vi "LVClass_HasoData dtor.vi"(0 "HasoData in":refnum<class "HasoData.lvclass">, 11 "error in (no error)":errorcluster) -> (4 "HasoData out":refnum<class "HasoData.lvclass">, 15 "error out":errorcluster)   [LabVIEW 2020, in "HasoData.lvclass"]
doc: "HasoData destructor.\n\n--------------------------------------------------------------------------------\n\n<B>HasoDataIn </B> : Pointer to HasoData object.\n<B>HasoDataOut </B> : Pointer to HasoData object.\n<B>ErrorIn </B> : Error\n<B>ErrorOut </B> : Error\n\n--------------------------------------------------------------------------------"
uses:
  HasoData.lvclass
  HasoData.lvclass/HasoData.ctl
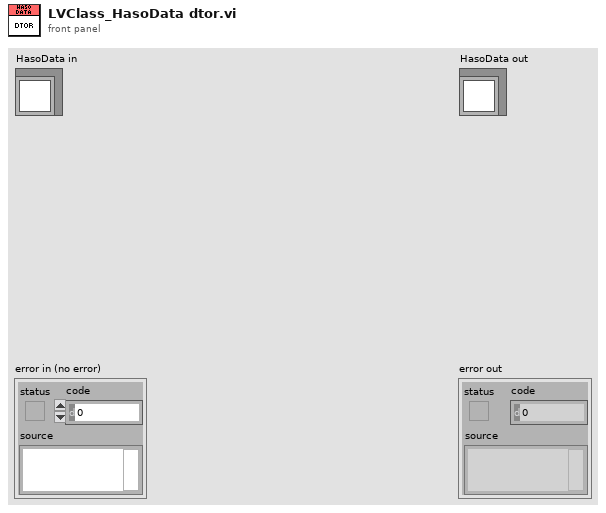
[diagram p1: front panel]
types:
  T1 = typedef "Handle creation.ctl" = enum16{"By ctor", "By write function"}
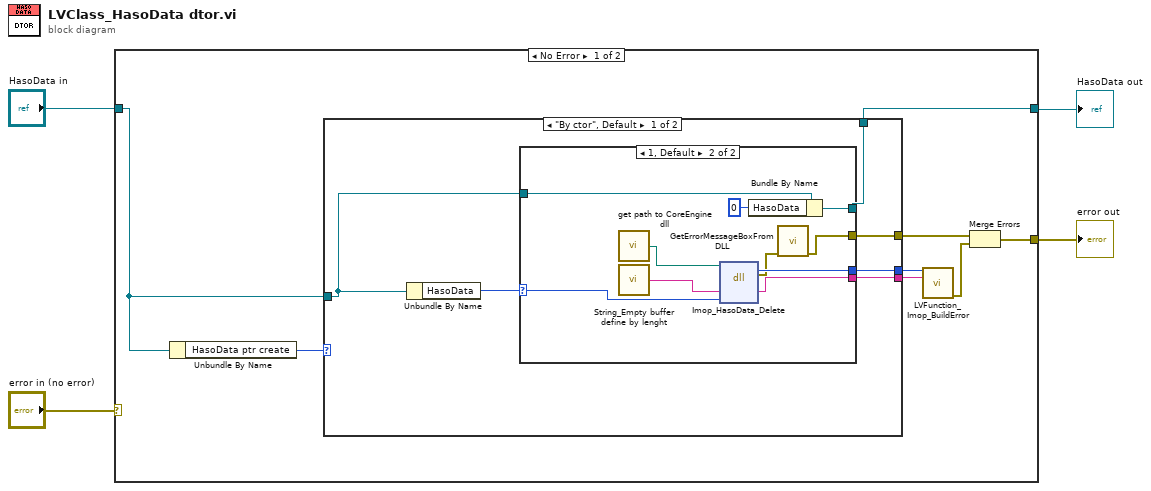
[diagram p0: block diagram]
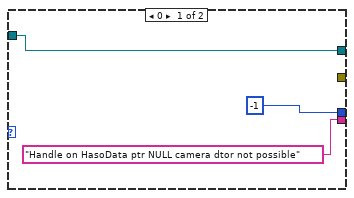
[diagram p2: hidden frame]
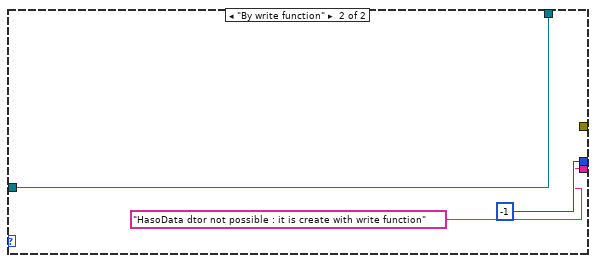
[diagram p3: hidden frame]
diagram:
  n1 = case shown="No Error" "error in (no error)" {
    selector: "error in (no error)" -> [_ w36]
    tunnel: [w5 w36] -> w1
    tunnel: [w10 w35] -> w2
    tunnel: "HasoData in" -> [w9 w35]
    frame No Error {
      n2 = Unbundle By Name(w9) -> ("HasoData ptr create"=w8:T1)
      n3 = case shown="\"By ctor\", Default" w8 {
        tunnel: [w18 "HasoData dtor not possible : it is create with write function" ("message")] -> w12
        tunnel: [w17 -1] -> w11
        tunnel: [w16 w34] -> w10
        tunnel: w9 -> [w15 w34]
        tunnel: [w13 _] -> w7
        frame "By ctor", Default {
          n4 = Unbundle By Name(w15) -> ("HasoData"=w14:i32)
          n5 = case shown="1, Default" w14 {
            selector: w14 -> [_ w28]
            tunnel: ["Handle on HasoData ptr NULL camera dtor not possible" ("message") w30] -> w18
            tunnel: [-1 w29] -> w17
            tunnel: [w19 w24] -> w16
            tunnel: w15 -> [w19 w23]
            tunnel: [_ w22] -> w13
            frame 0 {
            }
            frame 1, Default {
              n6 = call "get path to CoreEngine dll.vi"() -> ("path to c_interface_vc100.dll"=w27:path)  [unwired: 12 in, 3 out]
              n7 = call "String_Empty buffer define by lenght.vi"() -> ("Empty buffer"=w31:string)  [unwired: 1 in]
              n8 = dll-call lib="D:/soft/HASO_v3/SVN_trunk/ImOpCoreEngine4_LV2011/DLLs/c_interface_vc100.dll" fn="Imop_HasoData_Delete"(path in=w27, "message"=w31, "objet"=w28) -> (error out=w26:errorcluster, "return type"=w29:i32, "message"=w30:string)  [unwired: 3 in, 1 out]
              n9 = Bundle By Name(cluster=w23, "HasoData"=u32 0) -> (w24:refnum<class "HasoData.lvclass">)
              n10 = call "GetErrorMessageBoxFromDLL.vi"("error IN"=w26) -> ("error OUT"=w22:errorcluster)  [unwired: 10 in]
            }
          }
        }
        frame "By write function" {
        }
      }
      n11 = call "LVFunction_Imop_BuildError.vi"("code"=w11, "String to Prepend to source (\"\")"=w12) -> ("error out"=w6:errorcluster)  [unwired: 13 in]
      n12 = Merge Errors(w7, w6) -> (w5:errorcluster)
    }
    frame Error {
    }
  }
  "error out" <- w1
  "HasoData out" <- w2
